vi "parse_power_supply_reading.vi"(11 "read buffer 3":string) -> (0 "Current":dbl, 1 "Voltage":dbl, 2 "Current":string, 3 "Voltage":string)   [LabVIEW 2017]
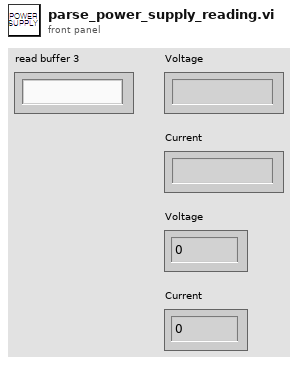
[diagram p1: front panel]
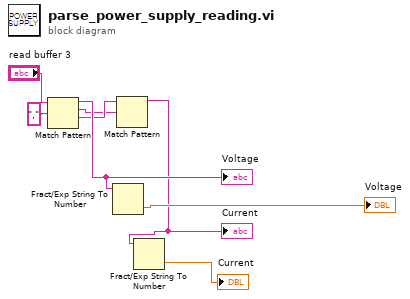
[diagram p0: block diagram]
diagram:
  n1 = Match Pattern(string="read buffer 3", regular expression=",") -> (before substring=w6:string, match substring=w4:string, after substring=w5:string)  [unwired: 1 in, 1 out]
  "Voltage" <- w6
  n2 = Fract/Exp String To Number(string=w6) -> (number=→"Voltage":dbl)  [unwired: 3 in, 1 out]
  n3 = Match Pattern(string=w5, regular expression=w4) -> (before substring=w1:string)  [unwired: 1 in, 3 out]
  "Current" <- w1
  n4 = Fract/Exp String To Number(string=w1) -> (number=→"Current":dbl)  [unwired: 3 in, 1 out]
